vi "PICO-500 Dishwasher 2023.vi"() -> ()   [LabVIEW 2015]
uses:
  <vilib>/userdefined/High Color/IMAQdx.ctl
  <vilib>/express/express signal manip/GetorSetDDTAttributes/Shared VIs/XDimension.ctl
  <vilib>/Utility/file.llb/Write Delimited Spreadsheet (string).vi
  <vilib>/express/express signal manip/GetorSetDDTAttributes/Shared VIs/XDimension Enum to String.vi
  <vilib>/express/express shared/transition.llb/Dynamic To Waveform Array.vi
  <vilib>/express/express signal manip/GetorSetDDTAttributes/Set DDT Attributes/SetT0.vi
  <vilib>/express/express shared/transition.llb/Waveform Array To Dynamic.vi
  <vilib>/express/express signal manip/GetorSetDDTAttributes/Set DDT Attributes/sub Set StartTimeStamp.vi
  <vilib>/FieldPoint/Polymorphic WriteRead.llb/FP WriteRead (Boolean).vi
  <vilib>/measure/mamon.llb/Waveform Peak Detection for 1 Chan.vi
  <vilib>/express/express signal manip/GetorSetDDTAttributes/Set DDT Attributes/Set DDT Properties.xnode
  <vilib>/vision/driver/NI_Vision_Acquisition_Software.lvlib
  <vilib>/express/express signal manip/GetorSetDDTAttributes/Shared VIs/GetSetShared.lvlib
  <vilib>/ptbypt/NI_PtbyPt.lvlib
  <vilib>/Analysis/NI_AALBase.lvlib
  <vilib>/express/express signal manip/GetorSetDDTAttributes/Set DDT Attributes/Set DDT Attributes.lvlib
  <vilib>/measure/NI_MAPro.lvlib
panel:
  out "Current File Path:":path caption="Filename Out"
  in  "Login Tab":enum32{"Login", "Data Aquisition"}(tab)
  in  "Login":bool
  in  "Select Surface":T1(radio)
  in  "Operator Name":string(combo)
  out "Path":path
  out "Live View":bool
  out "System Reset":bool
  in  "DAQ Tab":enum32{"General", "Plots", "Pressure Histogram"}(tab)
  in  "Heat Tape":bool
  in  "PD-25 (Circulation Pump)":bool
  in  "PD-26 (Drain Pump)":bool
  in  "Circulation Mode":bool
  in  "Begin Run":bool
  in  "Return to Login":bool
  out "Surface Selected":string
  in  "Nitrogen Flush Active?":bool
  out "Pressure":dynamicdata(graph)
  out "pH":dynamicdata(graph)
  out "Temperature":dynamicdata(graph)
  out "Heat Tape Circulation Out":dbl
  out "Heat Tape Circulation In":dbl
  out "Pressure Array":dbl[](array[numeric])
  out "Temperature Array":dbl[](array[numeric])
  out "pH Value":dbl
  out "Histogram of Pressure (PT-37)":T2(graph)
  out "Histogram of Pressure (PT-35)":T2(graph)
  out "?":T3(plugin-control)
  in  "Choose camera":T4
  in  "Close Camera":bool
  in  "Shutdown":bool
  out "Program Run-time":string caption="Elapsed Time Text"
  out "Circulation Run-Time":string caption="Elapsed Time Text"
  in  "Emergency Shutdown":bool
  # "PICO-500 Dishwasher DAQ V2.0\nUpdated Jan. 27, 2024"
  # "1. Click the \"Run\" Button - top left white arrow (Rightward facing) \n2. Select or type an operator from the list\n3. Select the Surface that will be cleaned\n4. Click \"Login\""
  # "Adding/Removing Operator:\n\n1. Before selecting \"Run\", right click the \"Operator Name\" string control box and select \"Edit Items\"\n\n2a. To add a new operator, select \"Insert\" and add the operator's name. Select \"ok\" when done.\n\n2b. To remove an operator, select \"Delete\". Select \"ok\" when done.\n\nOperator's name, surface selection, and other operations are recorded in the Activiy_Log.csv file when a new run is initiated."
  # "After Shutdown is complete, Click \"Abort Execution\" (Red Stop Sign Top Left)"
  # "-Nitrogen Flush must be confirmed and latched before \"RUN\" is activated\n-Click \"RUN\" to operate pumps and \"Circulation Mode\"\n-\"RUN\" will also enable live data aquisition and access to the remaining tabs. \"Run\" is active when highlighted green"
  # "Return To the login page. This will reset the current user configurations. \"Run\" must be disabled"
  # "Manual Control (For Adding/Removing cleaing solutions)"
  # "-Heat Tape will automatically turn on after 10 s\n-Heat tape upper limit is set to 200 C\n-Drain pump PD-26 is disabled in this mode\n-PD-25 will automatically run in this mode\n-Lower pressure limit set to 10 psi. When the average pressure reaches this value, the program cycles through the shutdown procedure."
  # "*Heat tape manual control is not recommended. *Heat tape will automatically turn on in circulation mode."
  # "PT-35 [Before Filtration]"
  # "PT-35 (Avg)"
  # "PT-37 [After Filtration]"
  # "PT-37 (Avg)"
  # "Pdiff_35_37 (Avg)"
  # "PT-39 [Pump Inlet]"
  # "PT-39 (Avg)"
  # "TT-38 [Inline Water Temp]"
  # "TT-40 [Ambient Temp]"
  # "TT-41 [Heat Tape Circ. Out]"
  # "TT-42 [Heat Tape Circ. In]"
  # "pH Value"
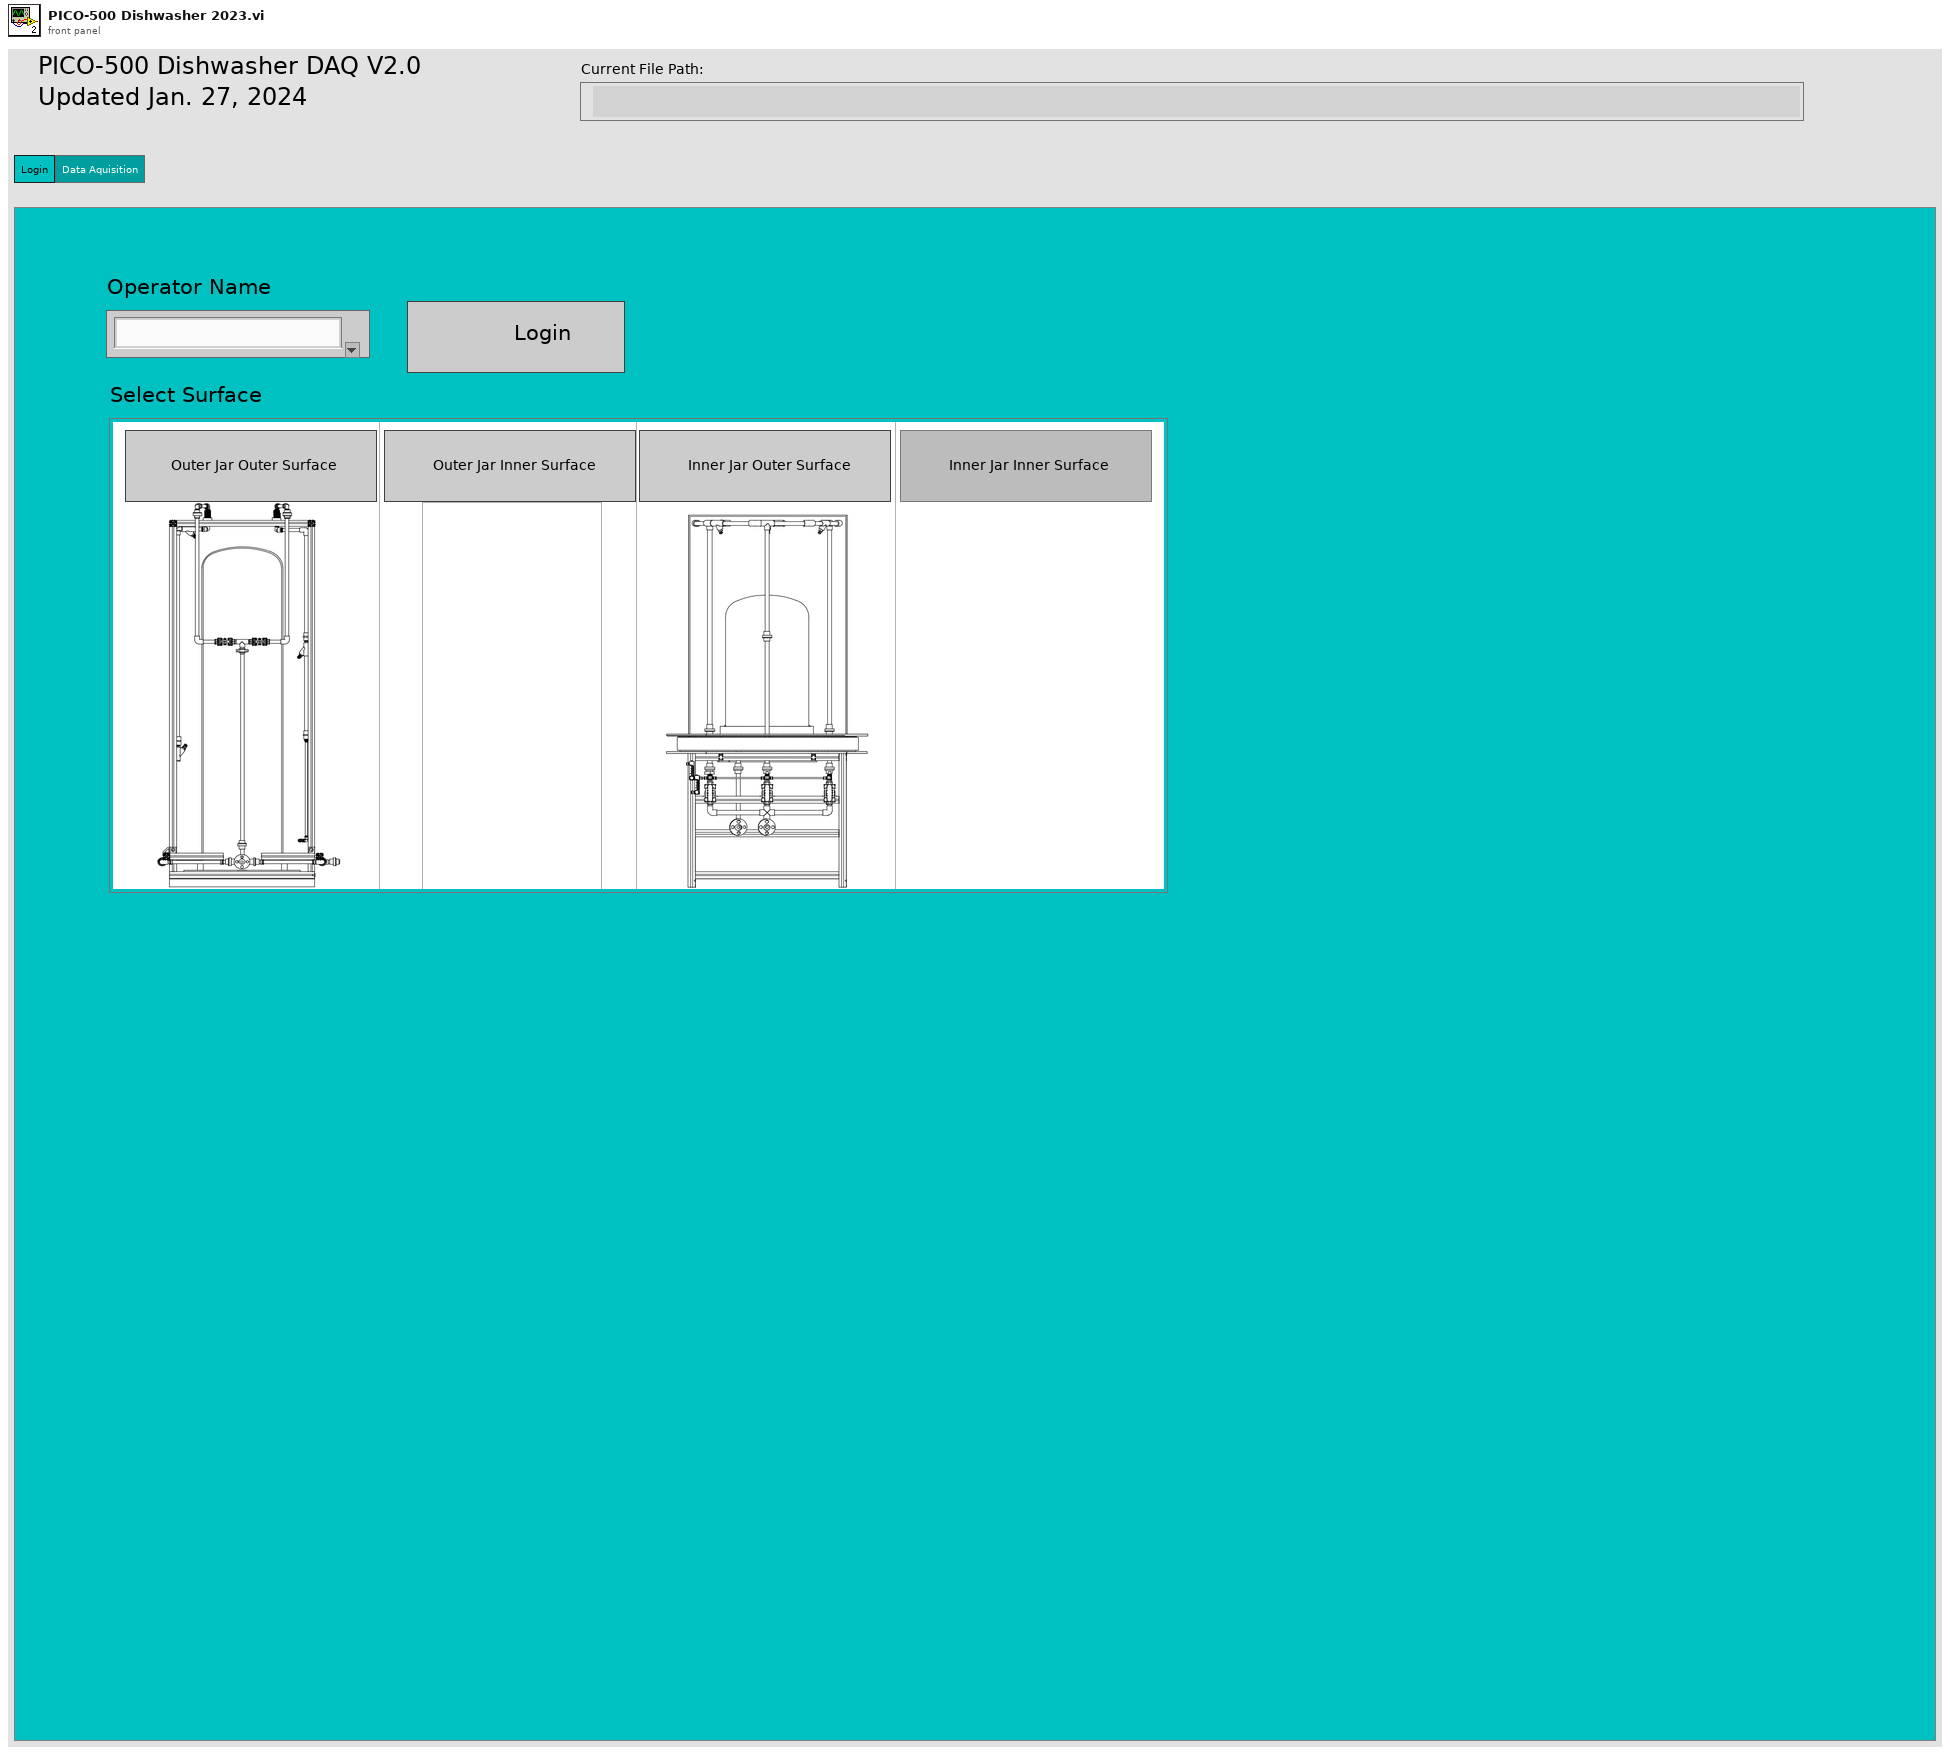
[diagram p1: front panel]
types:
  T1 = enum32{"No Selection", "Inner Jar Inner Surface", "Inner Jar Outer Surface", "Outer Jar Inner Surface", "Outer Jar Outer Surface"}
  T2 = cluster{"X Values":dbl[], "Histogram: h(x)":i32[]}
  T3 = typedef "IMAQ Image.ctl" = refnum<image>
  T4 = typedef "IMAQdx.ctl" = refnum<k21>
  T5 = enum16{"Start", "Login Page", "Go to DAQ", "Run DAQ", "Shutdown Heat Tape", "Shutdown Program", "Stop"}
  T6 = typedef "GetSetShared.lvlib/XDimension.ctl" = enum16{"No Unit [-]", "Time [sec]", "Frequency [Hz]"}
  T7 = cluster{dbl, "mean":dbl, dbl, "mean":dbl, dbl, dbl, "mean":dbl}
  T8 = typedef "Image Type" = u32
  T9 = enum32{"Page Enabled", "Page Disabled", "Page Disabled & Grayed"}
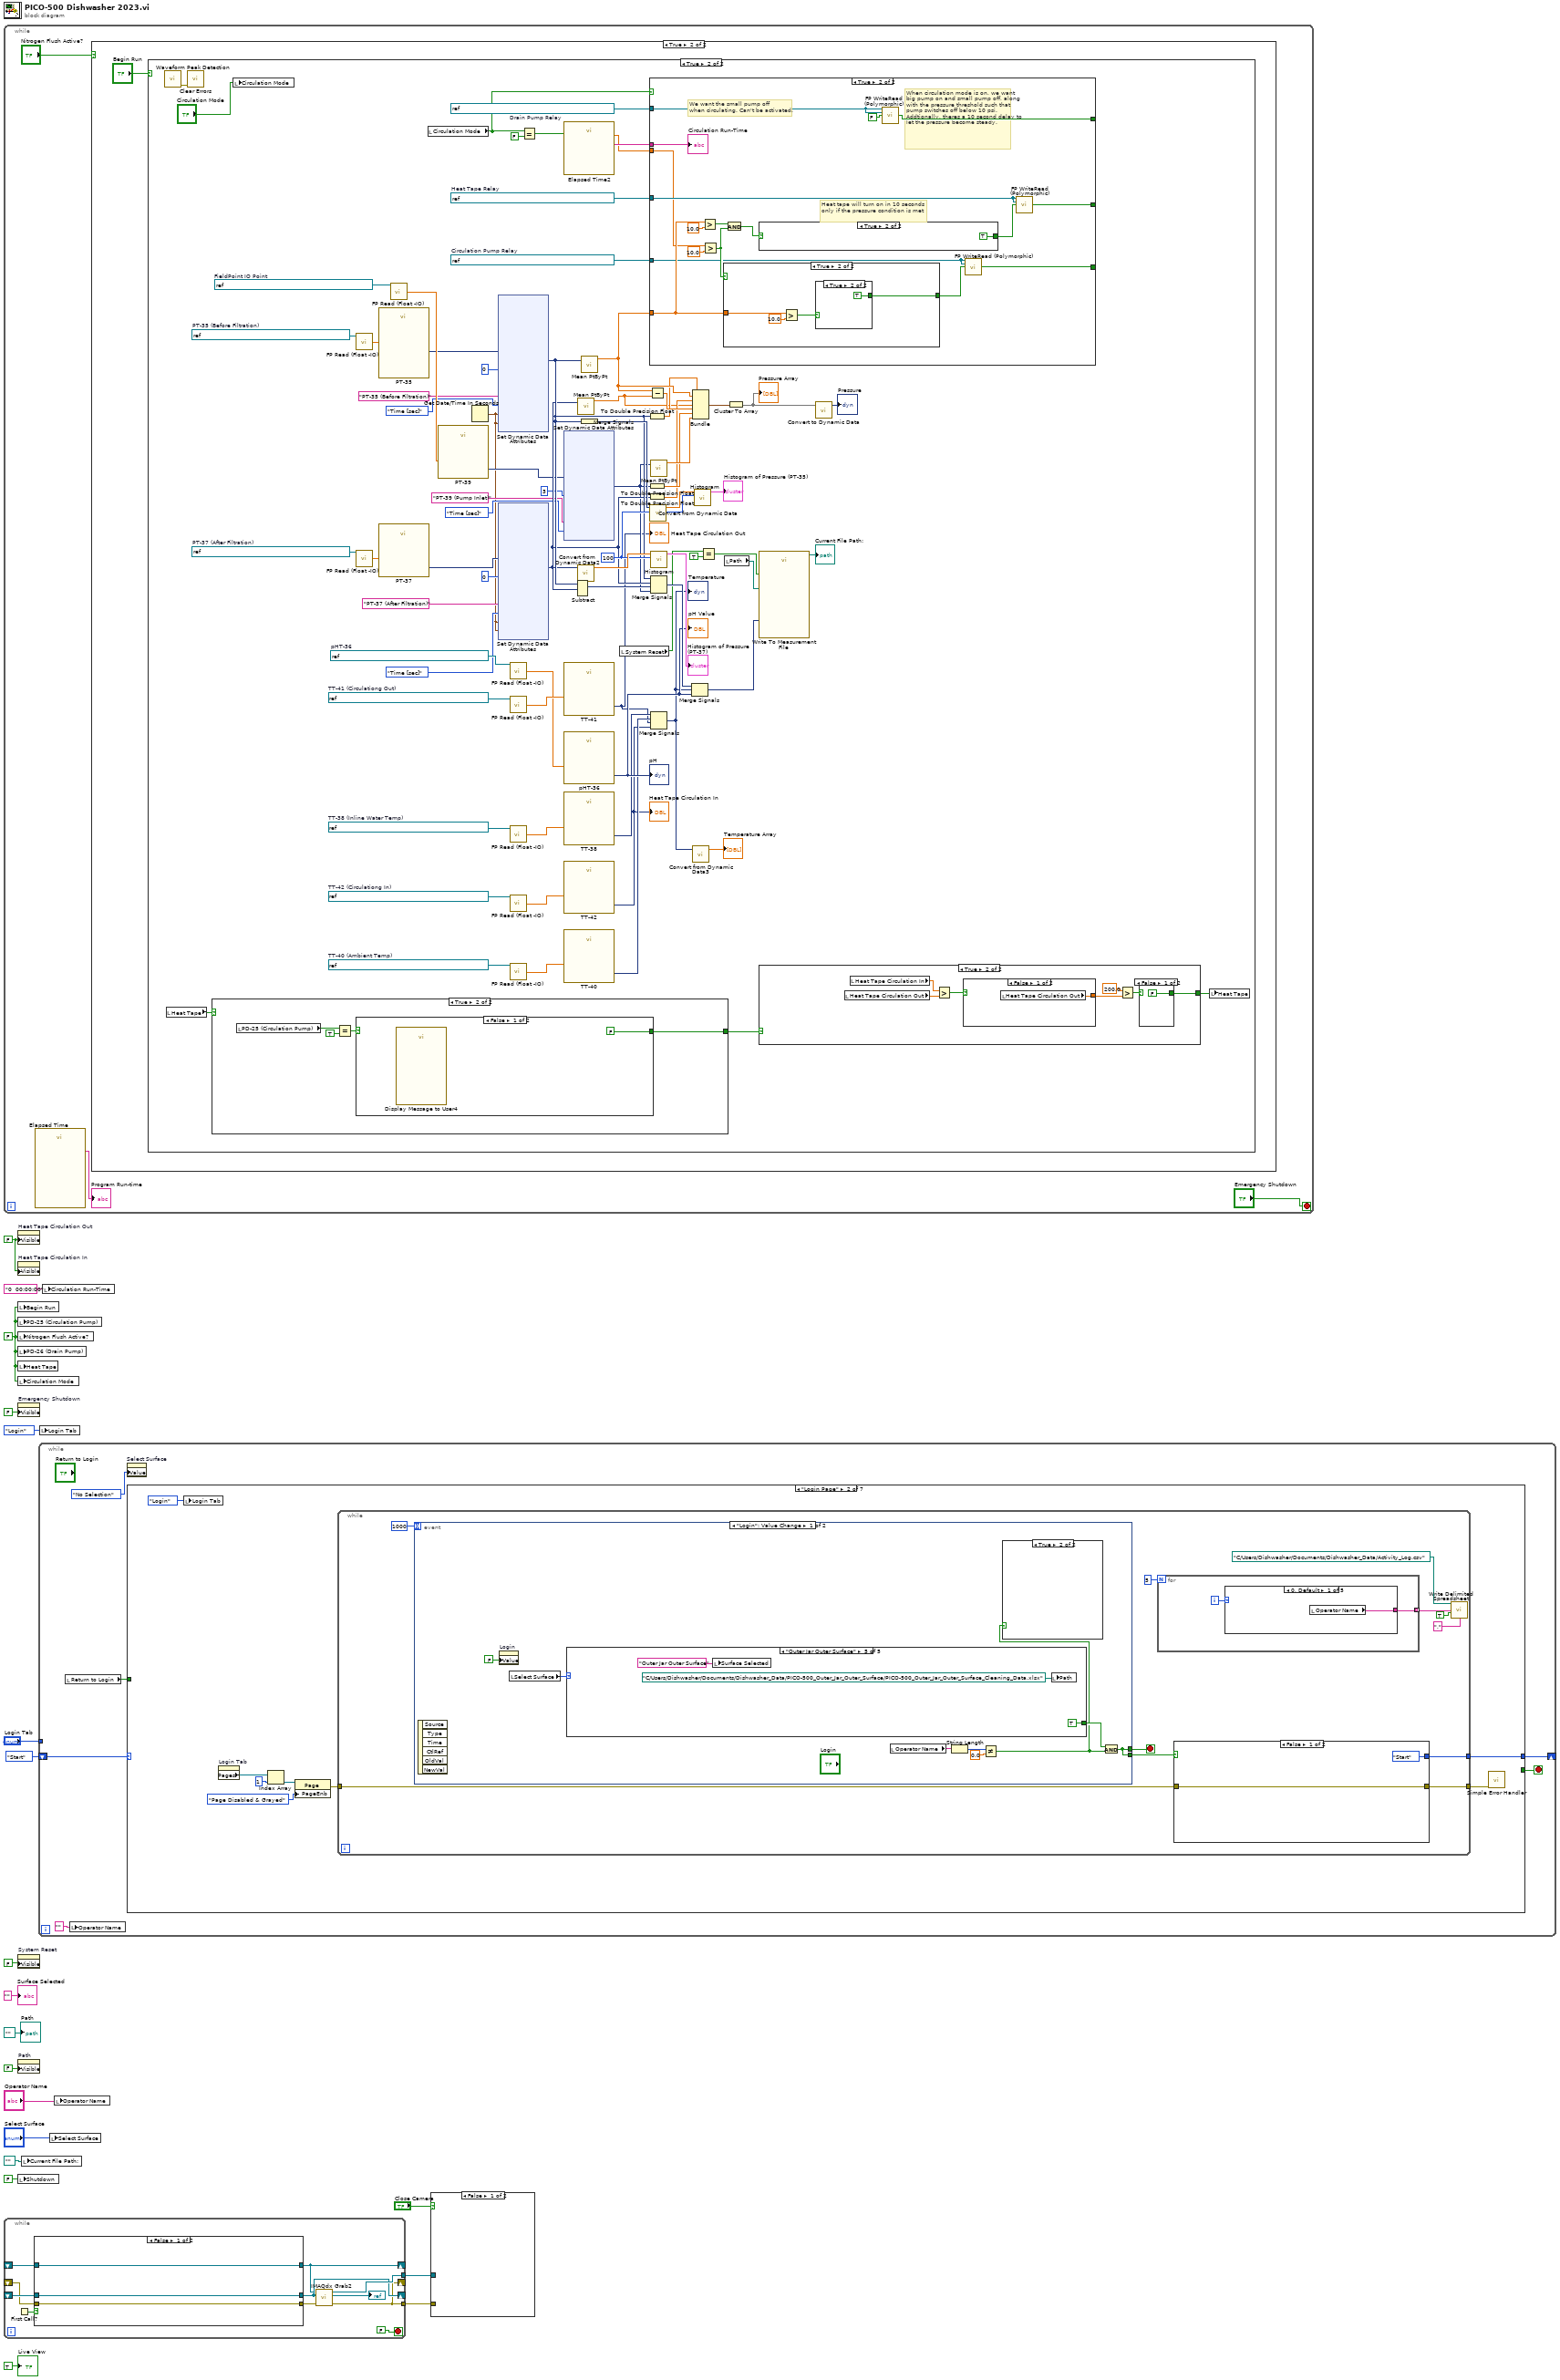
[diagram p0: block diagram]
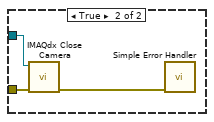
[diagram p2: hidden frame]
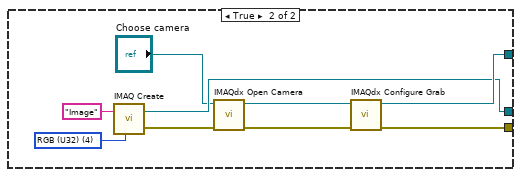
[diagram p3: hidden frame]
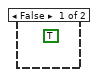
[diagram p5: hidden frame]
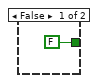
[diagram p6: hidden frame]
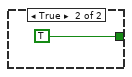
[diagram p7: hidden frame]
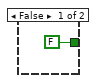
[diagram p8: hidden frame]
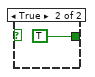
[diagram p9: hidden frame]
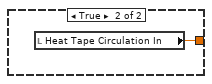
[diagram p10: hidden frame]
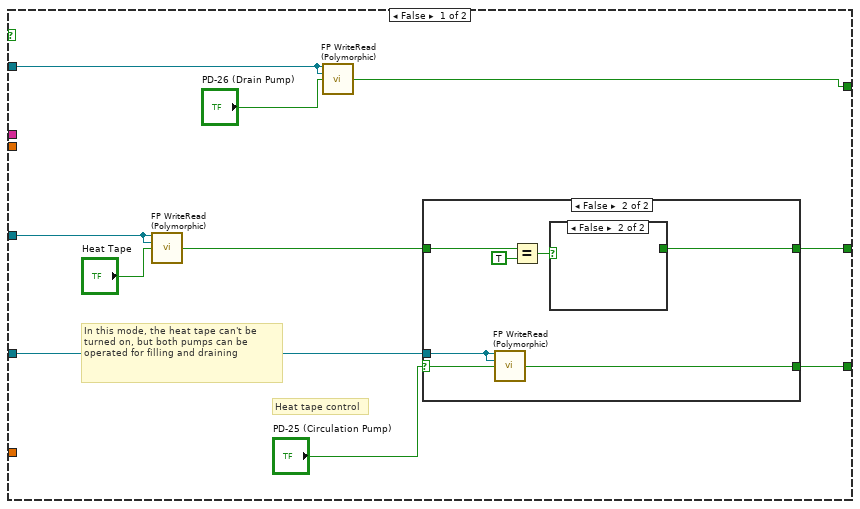
[diagram p11: hidden frame]
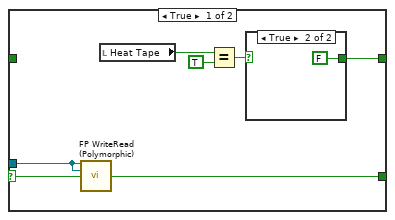
[diagram p12: hidden frame]
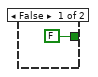
[diagram p13: hidden frame]
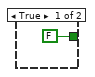
[diagram p14: hidden frame]
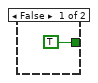
[diagram p15: hidden frame]
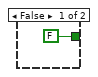
[diagram p16: hidden frame]
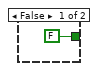
[diagram p17: hidden frame]
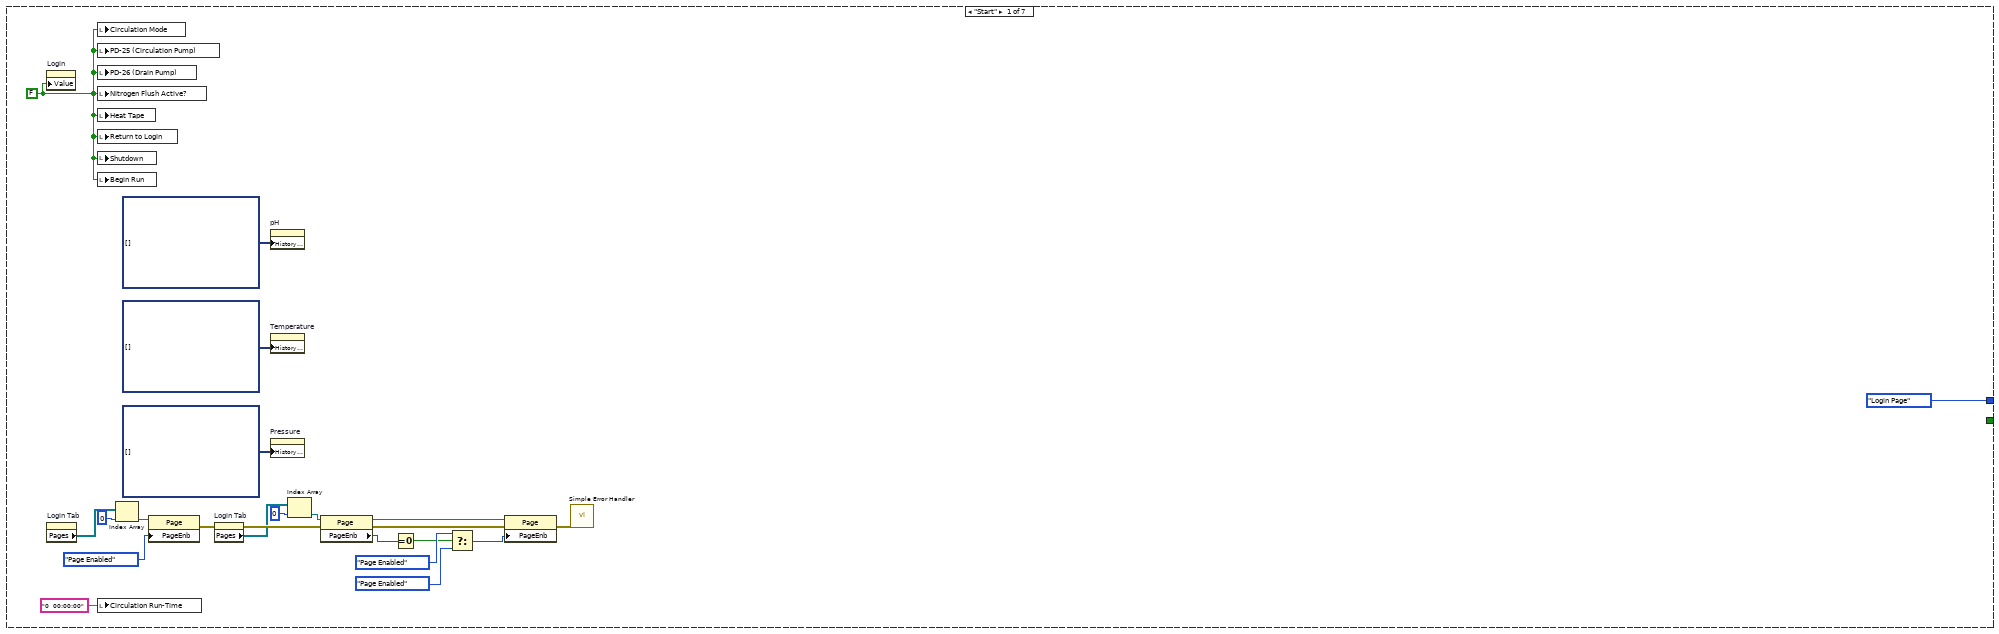
[diagram p18: hidden frame]
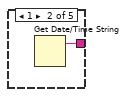
[diagram p19: hidden frame]
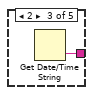
[diagram p20: hidden frame]
diagram:
  w9 = FALSE ("Visible")
  w7 = FALSE
  n1 = while {
    stop <- "Emergency Shutdown" stop-if-true
    n2 = call "Elapsed Time"() -> ("Elapsed Time Text"=→"Program Run-time":string)  [unwired: 12 in, 7 out]
    n3 = case shown="True" "Nitrogen Flush Active?" {
      frame False {
      }
      frame True {
        n4 = case shown="True" "Begin Run" {
          frame False {
            (unwired) TRUE
          }
          frame True {
            w56 = refnum<k21> "FieldPoint\\UofA-CPP-FP\\cFP-RLY-421 @3\\Channel 1"  # Circulation Pump Relay
            w61 = refnum<k21> "FieldPoint\\UofA-CPP-FP\\cFP-RLY-421 @3\\Channel 0"  # Drain Pump Relay
            w54 = refnum<k21> "FieldPoint\\UofA-CPP-FP\\cFP-RLY-421 @3\\Channel 2"  # Heat Tape Relay
            w78 = refnum<k21> "FieldPoint\\UofA-CPP-FP\\cFP-TC-120 @2\\Channel 3"  # TT-41 (Circulationg Out)
            w80 = 100
            w91 = refnum<k21> "FieldPoint\\UofA-CPP-FP\\cFP-TC-120 @2\\Channel 1"  # TT-42 (Circulationg In)
            w92 = refnum<k21> "FieldPoint\\UofA-CPP-FP\\cFP-AI-110 @1\\Channel 2"  # FieldPoint IO Point
            w94 = refnum<k21> "FieldPoint\\UofA-CPP-FP\\cFP-TC-120 @2\\Channel 0"  # TT-40 (Ambient Temp)
            w95 = refnum<k21> "FieldPoint\\UofA-CPP-FP\\cFP-TC-120 @2\\Channel 2"  # TT-38 (Inline Water Temp)
            w96 = refnum<k21> "FieldPoint\\UofA-CPP-FP\\cFP-AI-110 @1\\Channel 3"  # pHT-36
            w97 = refnum<k21> "FieldPoint\\UofA-CPP-FP\\cFP-AI-110 @1\\Channel 1"  # PT-35 (Before Filtration)
            w99 = refnum<k21> "FieldPoint\\UofA-CPP-FP\\cFP-AI-110 @1\\Channel 0"  # PT-37 (After Filtration)
            n5 = call-poly <vilib>:"Waveform Peak Detection.vi"() -> ("error out"=w40:errorcluster)  [unwired: 7 in, 4 out]
            n6 = local read "Heat Tape"() -> (w51:bool)
            n7 = call <vilib>:"Clear Errors.vi"("error in (no error)"=w40) -> ()  [unwired: 5 in, 2 out]
            n8 = case shown="True" w51 {
              tunnel: [FALSE w101] -> w53
              frame False {
              }
              frame True {
                n9 = local read "PD-25 (Circulation Pump)"() -> (w104:bool)
                n10 = Equal?(x=w104, y=TRUE) -> (x = y?=w102:bool)
                n11 = case shown="False" w102 {
                  tunnel: [FALSE TRUE] -> w101
                  frame False {
                    n12 = call "Display Message to User4"() -> ()  [unwired: 10 in, 2 out]
                  }
                  frame True {
                  }
                }
              }
            }
            n13 = local write "Circulation Mode"("Circulation Mode") -> ()
            n14 = call <vilib>:"FP Read (Float -IO).vi"("FieldPoint IO Point In"=w97) -> ("value"=w45:dbl)  [unwired: 11 in, 3 out]
            n15 = call <vilib>:"FP Read (Float -IO).vi"("FieldPoint IO Point In"=w99) -> ("value"=w98:dbl)  [unwired: 11 in, 3 out]
            n16 = call "PT-35"("Signals"=w45) -> ("Scaled Signals"=w43:dynamicdata)  [unwired: 9 in, 1 out]
            n17 = call "PT-37"("Signals"=w98) -> ("Scaled Signals"=w68:dynamicdata)  [unwired: 9 in, 1 out]
            n18 = call <vilib>:"FP Read (Float -IO).vi"("FieldPoint IO Point In"=w92) -> ("value"=w93:dbl)  [unwired: 11 in, 3 out]
            n19 = local read "Circulation Mode"() -> (w58:bool)
            n20 = call "PT-39"("Signals"=w93) -> ("Scaled Signals"=w63:dynamicdata)  [unwired: 9 in, 1 out]
            n21 = Get Date/Time In Seconds() -> (seconds since 1Jan1904=w41:timestamp)
            n22 = xnode "Set Dynamic Data Attributes"("Signals In"=w43, "Signal Index"=0, "Signal Name"="PT-35 (Before Filtration)", "X Dimension"=XDimension."Time [sec]", "Timestamp"=w41, "Start Timestamp"=w41) -> ("Signals Out"=w72:dynamicdata)  [unwired: 1 in, 1 out]
            n23 = xnode "Set Dynamic Data Attributes"("Signals In"=w68, "Signal Index"=0, "Signal Name"="PT-37 (After Filtration)", "X Dimension"=XDimension."Time [sec]", "Timestamp"=w41, "Start Timestamp"=w41) -> ("Signals Out"=w67:dynamicdata)  [unwired: 1 in, 1 out]
            n24 = call <vilib>:"FP Read (Float -IO).vi"("FieldPoint IO Point In"=w96) -> ("value"=w73:dbl)  [unwired: 11 in, 3 out]
            n25 = call <vilib>:"FP Read (Float -IO).vi"("FieldPoint IO Point In"=w78) -> ("value"=w77:dbl)  [unwired: 11 in, 3 out]
            n26 = call <vilib>:"FP Read (Float -IO).vi"("FieldPoint IO Point In"=w95) -> ("value"=w89:dbl)  [unwired: 11 in, 3 out]
            n27 = call <vilib>:"FP Read (Float -IO).vi"("FieldPoint IO Point In"=w91) -> ("value"=w90:dbl)  [unwired: 11 in, 3 out]
            n28 = call <vilib>:"FP Read (Float -IO).vi"("FieldPoint IO Point In"=w94) -> ("value"=w88:dbl)  [unwired: 11 in, 3 out]
            n29 = Equal?(x=w58, y=FALSE) -> (x = y?=w59:bool)
            n30 = call "Elapsed Time2"("Reset"=w59) -> ("Elapsed Time (s)"=w50:dbl, "Elapsed Time Text"=w55:string)  [unwired: 11 in, 6 out]
            n31 = xnode "Set Dynamic Data Attributes"("Signals In"=w63, "Signal Index"=3, "Signal Name"="PT-39 (Pump Inlet)", "X Dimension"=XDimension."Time [sec]") -> ("Signals Out"=w62:dynamicdata)  [unwired: 1 in, 1 out]
            n32 = call "TT-41"("Signals"=w77) -> ("Scaled Signals"=w32:dynamicdata)  [unwired: 9 in, 1 out]
            "Heat Tape Circulation Out" <- w32
            n33 = call "pHT-36"("Signals"=w73) -> ("Scaled Signals"=w81:dynamicdata)  [unwired: 9 in, 1 out]
            "pH" <- w81
            "pH Value" <- w81
            n34 = call "TT-38"("Signals"=w89) -> ("Scaled Signals"=w34:dynamicdata)  [unwired: 9 in, 1 out]
            n35 = call "TT-42"("Signals"=w90) -> ("Scaled Signals"=w31:dynamicdata)  [unwired: 9 in, 1 out]
            "Heat Tape Circulation In" <- w31
            n36 = call "TT-40"("Signals"=w88) -> ("Scaled Signals"=w33:dynamicdata)  [unwired: 9 in, 1 out]
            n37 = Subtract(1:w67, 2:w72) -> (0:w79:dynamicdata)  [unwired: 1 in, 1 out]
            n38 = call "Convert from Dynamic Data2"("Dynamic Data Type"=w67) -> ("Array"=w84:dbl[])  [unwired: 3 in]
            n39 = call <vilib>:"Mean PtByPt.vi"("x"=w67) -> ("mean"=w24:dbl)  [unwired: 3 in, 1 out]
            n40 = call <vilib>:"Mean PtByPt.vi"("x"=w72) -> ("mean"=w29:dbl)  [unwired: 3 in, 1 out]
            n41 = Merge Signals(w72) -> (w85:dynamicdata)
            n42 = local read "System Reset"() -> (w48:bool)
            n43 = case shown="True" w58 {
              tunnel: w29 -> [_ w154]
              tunnel: [w127 w161] -> _
              tunnel: [w124 w148] -> _
              tunnel: w61 -> [w125 w159]
              tunnel: w56 -> [w123 w152]
              tunnel: w54 -> [w120 w153]
              tunnel: [w122 w147] -> _
              tunnel: w50 -> [_ w149]
              tunnel: w55 -> [_ w146]
              frame False {
                # "Heat tape control"
                # "In this mode, the heat tape can't be turned on, but both pumps can be operated for filling and draining"
                n44 = call-poly <vilib>:"FP WriteRead (Polymorphic).vi"("FieldPoint Write Point"=w120, "FieldPoint Read Point"=w120, "value in"="Heat Tape") -> ("value out"=w119:bool)  [unwired: 10 in, 2 out]
                n45 = call-poly <vilib>:"FP WriteRead (Polymorphic).vi"("FieldPoint Write Point"=w125, "FieldPoint Read Point"=w125, "value in"="PD-26 (Drain Pump)") -> ("value out"=w127:bool)  [unwired: 10 in, 2 out]
                n46 = case shown="False" "PD-25 (Circulation Pump)" {
                  selector: "PD-25 (Circulation Pump)" -> [w134 w141]
                  tunnel: [w129 w142] -> w124
                  tunnel: w123 -> [w135 w139]
                  tunnel: [w133 w140] -> w122
                  tunnel: w119 -> [_ w138]
                  frame True {
                    n47 = call-poly <vilib>:"FP WriteRead (Polymorphic).vi"("FieldPoint Write Point"=w135, "FieldPoint Read Point"=w135, "value in"=w134) -> ("value out"=w133:bool)  [unwired: 10 in, 2 out]
                    n48 = local read "Heat Tape"() -> (w132:bool)
                    n49 = Equal?(x=w132, y=TRUE) -> (x = y?=w130:bool)
                    n50 = case shown="True" w130 {
                      tunnel: [FALSE FALSE] -> w129
                      frame False {
                      }
                      frame True {
                      }
                    }
                  }
                  frame False {
                    n51 = call-poly <vilib>:"FP WriteRead (Polymorphic).vi"("FieldPoint Write Point"=w139, "FieldPoint Read Point"=w139, "value in"=w141) -> ("value out"=w140:bool)  [unwired: 10 in, 2 out]
                    n52 = Equal?(x=w138, y=TRUE) -> (x = y?=w143:bool)
                    n53 = case shown="False" w143 {
                      tunnel: [FALSE _] -> w142
                      frame True {
                      }
                      frame False {
                      }
                    }
                  }
                }
              }
              frame True {
                # "Heat tape will turn on in 10 seconds only if the pressure condition is met"
                # "We want the small pump off\nwhen circulating. Can't be activated."
                # "When circulation mode is on, we want big pump on and small pump off, along with the pressure threshold such that pump switches off below 10 psi. Addtionally, theres a 10 second delay to let the pressure become steady."
                n54 = Greater?(x=w154, y=10.0 ("Pressure threshold ijo")) -> (0:w157:bool)
                n55 = Greater?(x=w149, y=10.0 ("Pressure threshold ijo")) -> (0:w155:bool)
                n56 = case shown="True" w155 {
                  tunnel: w154 -> [_ w166]
                  tunnel: [TRUE w164] -> w150
                  frame False {
                  }
                  frame True {
                    n57 = Greater?(x=w166, y=10.0 ("Pressure threshold ijo")) -> (0:w165:bool)
                    n58 = case shown="True" w165 {
                      tunnel: [FALSE TRUE] -> w164
                      frame False {
                      }
                      frame True {
                      }
                    }
                  }
                }
                n59 = And(x=w157, y=w155) -> (x .and. y?=w156:bool)
                n60 = case shown="True" w156 {
                  tunnel: [FALSE TRUE] -> w151
                  frame False {
                  }
                  frame True {
                  }
                }
                n61 = call-poly <vilib>:"FP WriteRead (Polymorphic).vi"("FieldPoint Write Point"=w159, "FieldPoint Read Point"=w159, "value in"=FALSE) -> ("value out"=w161:bool)  [unwired: 10 in, 2 out]
                n62 = call-poly <vilib>:"FP WriteRead (Polymorphic).vi"("FieldPoint Write Point"=w152, "FieldPoint Read Point"=w152, "value in"=w150) -> ("value out"=w147:bool)  [unwired: 10 in, 2 out]
                n63 = call-poly <vilib>:"FP WriteRead (Polymorphic).vi"("FieldPoint Write Point"=w153, "FieldPoint Read Point"=w153, "value in"=w151) -> ("value out"=w148:bool)  [unwired: 10 in, 2 out]
                "Circulation Run-Time" <- w146
              }
            }
            n64 = Subtract(x=w29, y=w24) -> (x-y=w30:dbl)
            n65 = To Double Precision Float(number=w72) -> (double precision float=w28:dbl)
            n66 = To Double Precision Float(number=w62) -> (double precision float=w26:dbl)
            n67 = To Double Precision Float(number=w67) -> (double precision float=w25:dbl)
            n68 = call "Convert from Dynamic Data"("Dynamic Data Type"=w85) -> ("Array"=w86:dbl[])  [unwired: 3 in]
            n69 = call <vilib>:"Mean PtByPt.vi"("x"=w62) -> ("mean"=w27:dbl)  [unwired: 3 in, 1 out]
            n70 = Merge Signals(w72, w67, w79, w62) -> (w82:dynamicdata)
            n71 = call <vilib>:"Histogram.vi"("intervals"=w80, "X"=w84) -> ("Histogram Graph"=→"Histogram of Pressure (PT-37)":T2)  [unwired: 6 in, 3 out]
            n72 = Merge Signals(w34, w33, w32, w31) -> (w35:dynamicdata)
            "Temperature" <- w35
            n73 = Merge Signals(w82, w35, w81) -> (w44:dynamicdata)
            n74 = Bundle(w28, "mean"=w29, w25, "mean"=w24, w30, w26, "mean"=w27) -> (w39:T7)  [unwired: 1 in]
            n75 = call "Convert from Dynamic Data3"("Dynamic Data Type"=w35) -> ("Array"=→"Temperature Array":dbl[])  [unwired: 3 in]
            n76 = call <vilib>:"Histogram.vi"("intervals"=w80, "X"=w86) -> ("Histogram Graph"=→"Histogram of Pressure (PT-35)":T2)  [unwired: 6 in, 3 out]
            n77 = Equal?(x=w48, y=TRUE) -> (x = y?=w46:bool)
            n78 = local read "Path"() -> (w42:path)
            n79 = Cluster To Array(cluster=w39) -> (array=w38:dbl[])
            "Pressure Array" <- w38
            n80 = call "Write To Measurement File"("Signals"=w44, "new_file"=w46, "Filename"=w42) -> ("Filename Out"=→"Current File Path:":path)  [unwired: 14 in, 2 out]
            n81 = case shown="True" w53 {
              tunnel: [FALSE w114] -> w52
              frame False {
              }
              frame True {
                n82 = local read "Heat Tape Circulation Out"() -> (w109:dbl)
                n83 = local read "Heat Tape Circulation In"() -> (w110:dbl)
                n84 = Greater?(x=w110, y=w109) -> (0:w113:bool)
                n85 = case shown="False" w113 {
                  tunnel: [w117 w118] -> w108
                  frame False {
                    n86 = local read "Heat Tape Circulation Out"() -> (w117:dbl)
                  }
                  frame True {
                    n87 = local read "Heat Tape Circulation In"() -> (w118:dbl)
                  }
                }
                n88 = Greater?(x=200.0, y=w108) -> (0:w112:bool)
                n89 = case shown="False" w112 {
                  tunnel: [FALSE TRUE] -> w114
                  frame False {
                  }
                  frame True {
                  }
                }
              }
            }
            n90 = call "Convert to Dynamic Data"("Array"=w38) -> ("Dynamic Data Type"=→"Pressure":dynamicdata)  [unwired: 3 in]
            n91 = local write "Heat Tape"(w52) -> ()
          }
        }
      }
    }
  }
  n92 = while {
    tunnel: [w250] -> w4
    tunnel: [w243] -> w3
    shift-right: [w247] -> _
    shift-left: _ -> [w246]
    shift-right: [w245] -> _
    shift-left: _ -> [w244]
    shift-right: [w243] -> _
    shift-left: _ -> [w242]
    stop <- FALSE stop-if-true
    n93 = First Call?() -> (First Call?: T/F=w248:bool)
    n94 = case shown="False" w248 {
      tunnel: [w252 w261] -> w245
      tunnel: [w251 w259] -> w249
      tunnel: [w253 w256] -> w247
      tunnel: w246 -> [w253 _]
      tunnel: w244 -> [w252 _]
      tunnel: w242 -> [w251 _]
      frame False {
      }
      frame True {
        w257 = T8 4 items=["Grayscale (U8)", "Grayscale (I16)", "Grayscale (SGL)", "Complex (CSG)", "RGB (U32)", "HSL (U32)", "RGB (U64)", "Grayscale (U16)"] ("Image Type")
        n95 = call "IMAQ Create"("Image Name"="Image", "Image Type"=w257) -> ("New Image"=w256:T3, "error out"=w255:errorcluster)  [unwired: 3 in]
        n96 = call <vilib>:"IMAQdx Open Camera.vi"("error in"=w255, "Session In"="Choose camera") -> ("error out"=w260:errorcluster, "Session Out"=w262:T4)  [unwired: 8 in]
        n97 = call <vilib>:"IMAQdx Configure Grab.vi"("error in"=w260, "Session In"=w262) -> ("error out"=w259:errorcluster, "Session Out"=w261:T4)  [unwired: 8 in]
      }
    }
    n98 = call <vilib>:"IMAQdx Grab2.vi"("error in"=w249, "Image In"=w247, "Session In"=w245) -> ("error out"=w243:errorcluster, "Image Out"=→"?":T3, "Session Out"=w250:T4)  [unwired: 5 in, 1 out]
  }
  n99 = property on="Heat Tape Circulation Out" class="DigNum (strict)"("Visible"=w9) -> ()  [unwired: 2 in, 2 out]
  n100 = property on="Heat Tape Circulation In" class="DigNum (strict)"("Visible"=w9) -> ()  [unwired: 2 in, 2 out]
  n101 = local write "Begin Run"(w7) -> ()
  n102 = local write "PD-25 (Circulation Pump)"(w7) -> ()
  n103 = local write "Nitrogen Flush Active?"(w7) -> ()
  n104 = local write "PD-26 (Drain Pump)"(w7) -> ()
  n105 = local write "Heat Tape"(w7) -> ()
  n106 = local write "Circulation Mode"(w7) -> ()
  n107 = property on="Emergency Shutdown" class="Bool (strict)"("Visible"=FALSE) -> ()  [unwired: 2 in, 2 out]
  n108 = property on="System Reset" class="Bool (strict)"("Visible"=FALSE) -> ()  [unwired: 2 in, 2 out]
  n109 = property on="Path" class="Path"("Visible"=FALSE) -> ()  [unwired: 2 in, 2 out]
  n110 = local write "Shutdown"(FALSE) -> ()
  n111 = local write "Current File Path:"(path "" ("Current File Path:")) -> ()
  n112 = while {
    shift-right: [w267] -> _
    shift-left: T5."Start" -> [w268]
    tunnel: "Login Tab" -> [_]
    stop <- w266 stop-if-true
    n113 = local read "Return to Login"() -> (w263:bool)
    n114 = local write "Operator Name"("") -> ()
    n115 = property on="Select Surface" class="RadioBtnsControl (strict)"("Value"=T1."No Selection" ("Select Surface")) -> ()  [unwired: 2 in, 2 out]
    n116 = case shown="\"Login Page\"" w268 {
      tunnel: [T5."Login Page" w293 T5."Run DAQ" w388 T5."Shutdown Program" w411 T5."Stop"] -> w267
      tunnel: [_ _ _ _ _ _ TRUE] -> w266
      tunnel: w263 -> [_ _ _ w387 _ _ _]
      frame "Start" {
        w271 = FALSE ("Begin Run")
        n117 = property on="Login" class="Bool (strict)"("Value"=w271) -> ()  [unwired: 2 in, 2 out]
        n118 = property on="Login Tab" class="TabCtl (strict)"() -> ("Pages"=w288:refnum<vi>[])  [unwired: 2 in, 2 out]
        n119 = local write "Circulation Mode"(w271) -> ()
        n120 = local write "PD-25 (Circulation Pump)"(w271) -> ()
        n121 = local write "PD-26 (Drain Pump)"(w271) -> ()
        n122 = local write "Nitrogen Flush Active?"(w271) -> ()
        n123 = local write "Heat Tape"(w271) -> ()
        n124 = local write "Return to Login"(w271) -> ()
        n125 = local write "Shutdown"(w271) -> ()
        n126 = local write "Begin Run"(w271) -> ()
        n127 = local write "Circulation Run-Time"("0  00:00:00" ("Circulation Run-Time")) -> ()
        n128 = Index Array(array=w288, index=0) -> (element=w290:refnum<vi>)
        n129 = property class="Page"(reference=w290, "PageEnb"=T9."Page Enabled" ("Page Enabled State")) -> (error out=w276:errorcluster)  [unwired: 1 in, 1 out]
        n130 = property on="Login Tab" class="TabCtl (strict)"(error in=w276) -> (error out=w286:errorcluster, "Pages"=w277:refnum<vi>[])  [unwired: 1 in, 1 out]
        n131 = property on="pH" class="WFChart (strict)"("History Data"=dynamicdata[] []) -> ()  [unwired: 2 in, 2 out]
        n132 = property on="Temperature" class="WFChart (strict)"("History Data"=dynamicdata[] []) -> ()  [unwired: 2 in, 2 out]
        n133 = property on="Pressure" class="WFChart (strict)"("History Data"=dynamicdata[] []) -> ()  [unwired: 2 in, 2 out]
        n134 = Index Array(array=w277, index=0) -> (element=w279:refnum<vi>)
        n135 = property class="Page"(reference=w279, error in=w286) -> (reference out=w280:refnum<vi>, error out=w287:errorcluster, "PageEnb"=w281:T9)
        n136 = Equal To 0?(x=w281) -> (x = 0?=w282:bool)
        n137 = Select(t=T9."Page Enabled" ("Page Enabled State"), s=w282, f=T9."Page Enabled" ("Page Enabled State")) -> (s? t:f=w285:T9)
        n138 = property class="Page"(reference=w280, error in=w287, "PageEnb"=w285) -> (error out=w275:errorcluster)  [unwired: 1 out]
        n139 = call <vilib>:"Simple Error Handler.vi"("error in (no error)"=w275) -> ()  [unwired: 4 in, 5 out]
      }
      frame "Login Page" {
        n140 = local write "Login Tab"(enum32{"Login", "Data Aquisition"}."Login" ("Tab Control 3")) -> ()
        n141 = property on="Login Tab" class="TabCtl (strict)"() -> ("Pages"=w294:refnum<vi>[])  [unwired: 2 in, 2 out]
        n142 = Index Array(array=w294, index=1) -> (element=w296:refnum<vi>)
        n143 = property class="Page"(reference=w296, "PageEnb"=T9."Page Disabled & Grayed" ("Page Enabled State")) -> (error out=w298:errorcluster)  [unwired: 1 in, 1 out]
        n144 = while {
          tunnel: w298 -> [w309]
          tunnel: [w308] -> w299
          tunnel: [w306] -> w293
          stop <- w310 stop-if-true
          n145 = event shown="[0] \"Login\": Value Change" {
            selector: _ -> [_ _]
            dyn-events: _ -> [_ _]
            timeout: 1000 -> [_ _]
            tunnel: [w339 _] -> w310
            tunnel: [w339 _] -> w307
            event "Login": Value Change {
              n146 = event-data() -> ()  [unwired: 1 in, 6 out]
              n147 = property on="Login" class="Bool (strict)"("Value"=FALSE ("Login")) -> ()  [unwired: 2 in, 2 out]
              n148 = local read "Select Surface"() -> (w341:T1)
              n149 = case shown="\"Outer Jar Outer Surface\"" w341 {
                tunnel: [FALSE TRUE TRUE TRUE TRUE] -> w340
                frame "No Selection", Default {
                  n150 = call "Display Message to User3"() -> ()  [unwired: 10 in, 2 out]
                }
                frame "Inner Jar Inner Surface" {
                  n151 = local write "Surface Selected"("Inner Jar Inner Surface") -> ()
                  n152 = local write "Path"(path "C:/Users/Dishwasher/Documents/Dishwasher_Data/PICO-500_Inner_Jar_Inner_Surface/PICO-500_Inner_Jar_Inner_Surface_Cleaning_Data.xlsx" ("Path")) -> ()
                }
                frame "Inner Jar Outer Surface" {
                  n153 = local write "Surface Selected"("Inner Jar Outer Surface") -> ()
                  n154 = local write "Path"(path "C:/Users/Dishwasher/Documents/Dishwasher_Data/PICO-500_Inner_Jar_Outer_Surface/PICO-500_Inner_Jar_Outer_Surface_Cleaning_Data.xlsx" ("Path")) -> ()
                }
                frame "Outer Jar Inner Surface" {
                  n155 = local write "Surface Selected"("Outer Jar Inner Surface") -> ()
                  n156 = local write "Path"(path "C:/Users/Dishwasher/Documents/Dishwasher_Data/PICO-500_Outer_Jar_Inner_Surface/PICO-500_Outer_Jar_Inner_Surface_Cleaning_Data.xlsx" ("Path")) -> ()
                }
                frame "Outer Jar Outer Surface" {
                  n157 = local write "Surface Selected"("Outer Jar Outer Surface") -> ()
                  n158 = local write "Path"(path "C:/Users/Dishwasher/Documents/Dishwasher_Data/PICO-500_Outer_Jar_Outer_Surface/PICO-500_Outer_Jar_Outer_Surface_Cleaning_Data.xlsx" ("Path")) -> ()
                }
              }
              n159 = local read "Operator Name"() -> (w335:string)
              n160 = String Length(string=w335) -> (length=w337:i32)
              n161 = Not Equal?(x=w337, y=0.0) -> (x != y?=w336:bool)
              n162 = case shown="True" w336 {
                frame False {
                  n163 = call "Display Message to User2"() -> ()  [unwired: 10 in, 2 out]
                }
                frame True {
                }
              }
              n164 = And(x=w340, y=w336) -> (x .and. y?=w339:bool)
            }
            event Timeout {
              n165 = event-data() -> ()  [unwired: 1 in, 3 out]
            }
          }
          n166 = for {
            N: 5 -> [_]
            tunnel: [w311] -> w302 mode=indexing
            i -> [w312]
            n167 = case shown="0, Default" w312 {
              tunnel: [w313 w314 w315 w316 "Starting the LabVIEW program"] -> w311
              frame 0, Default {
                n168 = local read "Operator Name"() -> (w313:string)
              }
              frame 1 {
                n169 = Get Date/Time String() -> (date string=w314:string)  [unwired: 3 in, 1 out]
              }
              frame 2 {
                n170 = Get Date/Time String() -> (time string=w315:string)  [unwired: 3 in, 1 out]
              }
              frame 4 {
                n171 = local read "Surface Selected"() -> (w316:string)
              }
              frame 3 {
              }
            }
          }
          n172 = case shown="False" w307 {
            tunnel: w309 -> [w319 w331]
            tunnel: [w319 w323] -> w308
            tunnel: [T5."Start" T5."Go to DAQ"] -> w306
            frame False {
            }
            frame True {
              n173 = property on="Login Tab" class="TabCtl (strict)"(error in=w331) -> (error out=w322:errorcluster, "Pages"=w333:refnum<vi>[])  [unwired: 1 in, 1 out]
              n174 = Index Array(array=w333, index=1) -> (element=w330:refnum<vi>)
              n175 = property class="Page"(reference=w330, error in=w322) -> (reference out=w329:refnum<vi>, error out=w321:errorcluster, "PageEnb"=w328:T9)
              n176 = Equal To 0?(x=w328) -> (x = 0?=w327:bool)
              n177 = Select(t=T9."Page Disabled & Grayed" ("Page Enabled State"), s=w327, f=T9."Page Enabled" ("Page Enabled State")) -> (s? t:f=w324:T9)
              n178 = property class="Page"(reference=w329, error in=w321, "PageEnb"=w324) -> (error out=w323:errorcluster)  [unwired: 1 out]
            }
          }
          n179 = call-poly <vilib>:"Write Delimited Spreadsheet.vi"("file path (dialog if empty)"=path "C:/Users/Dishwasher/Documents/Dishwasher_Data/Activity_Log.csv", "1D data"=w302, "append to file? (F)"=TRUE, "delimiter (\\t)"="," ("delimiter (\\t)")) -> ()  [unwired: 10 in, 2 out]
        }
        n180 = call <vilib>:"Simple Error Handler.vi"("error in (no error)"=w299) -> ()  [unwired: 4 in, 5 out]
      }
      frame "Go to DAQ" {
        n181 = Wait (ms)(milliseconds to wait=u32 50) -> ()  [unwired: 1 out]
        n182 = local write "DAQ Tab"(enum32{"General", "Plots", "Pressure Histogram"}."General" ("DAQ Tab")) -> ()
        n183 = property on="Login Tab" class="TabCtl (strict)"() -> ("Pages"=w362:refnum<vi>[])  [unwired: 2 in, 2 out]
        n184 = local write "Login Tab"(enum32{"Login", "Data Aquisition"}."Data Aquisition" ("Tab Control 3")) -> ()
        n185 = Index Array(array=w362, index=0) -> (element=w364:refnum<vi>)
        n186 = local read "Shutdown"() -> (w359:bool)
        n187 = property class="Page"(reference=w364, "PageEnb"=T9."Page Disabled & Grayed" ("Page Enabled State")) -> (error out=w360:errorcluster)  [unwired: 1 in, 1 out]
        n188 = case shown="False" w359 {
          tunnel: [w366 w368] -> w361
          tunnel: w360 -> [w366 w367]
          frame False {
          }
          frame True {
            n189 = property on="Login Tab" class="TabCtl (strict)"(error in=w367) -> (error out=w378:errorcluster, "Pages"=w369:refnum<vi>[])  [unwired: 1 in, 1 out]
            n190 = Index Array(array=w369, index=0) -> (element=w371:refnum<vi>)
            n191 = property class="Page"(reference=w371, error in=w378) -> (reference out=w372:refnum<vi>, error out=w379:errorcluster, "PageEnb"=w373:T9)
            n192 = Equal To 0?(x=w373) -> (x = 0?=w374:bool)
            n193 = Select(t=T9."Page Disabled & Grayed" ("Page Enabled State"), s=w374, f=T9."Page Enabled" ("Page Enabled State")) -> (s? t:f=w377:T9)
            n194 = property class="Page"(reference=w372, error in=w379, "PageEnb"=w377) -> (error out=w368:errorcluster)  [unwired: 1 out]
          }
        }
        n195 = call <vilib>:"Simple Error Handler.vi"("error in (no error)"=w361) -> ()  [unwired: 4 in, 5 out]
      }
      frame "Run DAQ" {
        n196 = case shown="False" w387 {
          tunnel: [w392 w400] -> w388
          frame False {
            n197 = local read "Begin Run"() -> (w391:bool)
            n198 = case shown="True" w391 {
              tunnel: [T5."Go to DAQ" T5."Run DAQ"] -> w394
              frame False {
                n199 = local write "System Reset"(TRUE) -> ()
              }
              frame True {
                n200 = local write "System Reset"(FALSE) -> ()
              }
            }
            n201 = Select(t=T5."Shutdown Heat Tape", s="Shutdown", f=w394) -> (s? t:f=w392:T5)
          }
          frame True {
            n202 = local read "Begin Run"() -> (w399:bool)
            n203 = case shown="False" w399 {
              tunnel: [T5."Start" T5."Run DAQ"] -> w400
              frame False {
                n204 = local write "Heat Tape"(FALSE) -> ()
                n205 = local write "Circulation Mode"(FALSE) -> ()
                n206 = local write "PD-25 (Circulation Pump)"(FALSE) -> ()
                n207 = local write "PD-26 (Drain Pump)"(FALSE) -> ()
                "System Reset" <- FALSE
              }
              frame True {
                n208 = call "Display Message to User"() -> ()  [unwired: 10 in, 2 out]
              }
            }
          }
        }
        n209 = local read "Nitrogen Flush Active?"() -> (w386:bool)
        n210 = local read "Begin Run"() -> (w384:bool)
        n211 = Equal?(x=w386, y=FALSE) -> (x = y?=w382:bool)
        n212 = Equal?(x=w384, y=TRUE) -> (x = y?=w381:bool)
        n213 = And(x=w382, y=w381) -> (x .and. y?=w380:bool)
        n214 = case shown="True" w380 {
          frame False {
          }
          frame True {
            n215 = call "Display Message to User5"() -> ()  [unwired: 10 in, 2 out]
            n216 = local write "Begin Run"(FALSE) -> ()
          }
        }
      }
      frame "Shutdown Heat Tape" {
        n217 = local write "Heat Tape"(FALSE) -> ()
        n218 = local write "Circulation Mode"(FALSE) -> ()
      }
      frame "Shutdown Program" {
        w416 = 80.0 ("y")
        n219 = local read "Heat Tape Circulation Out"() -> (w415:dbl)
        n220 = local read "Heat Tape Circulation In"() -> (w417:dbl)
        n221 = Greater?(x=w417, y=w416) -> (0:w413:bool)
        n222 = Greater?(x=w415, y=w416) -> (0:w414:bool)
        n223 = Or(x=w413, y=w414) -> (x .or. y?=w412:bool)
        n224 = case shown="True" w412 {
          tunnel: [T5."Stop" T5."Shutdown Program"] -> w411
          frame False {
            n225 = local write "PD-25 (Circulation Pump)"(FALSE) -> ()
          }
          frame True {
            n226 = local write "PD-25 (Circulation Pump)"(TRUE) -> ()
          }
        }
      }
      frame "Stop" {
        n227 = local write "Emergency Shutdown"(TRUE) -> ()
        n228 = local write "Begin Run"(FALSE) -> ()
        n229 = property on="Login Tab" class="TabCtl (strict)"() -> ("Pages"=w438:refnum<vi>[])  [unwired: 2 in, 2 out]
        n230 = Index Array(array=w438, index=0) -> (element=w440:refnum<vi>)
        n231 = property class="Page"(reference=w440, "PageEnb"=T9."Page Enabled" ("Page Enabled State")) -> (error out=w426:errorcluster)  [unwired: 1 in, 1 out]
        n232 = property on="Login Tab" class="TabCtl (strict)"(error in=w426) -> (error out=w436:errorcluster, "Pages"=w427:refnum<vi>[])  [unwired: 1 in, 1 out]
        n233 = Index Array(array=w427, index=0) -> (element=w429:refnum<vi>)
        n234 = property class="Page"(reference=w429, error in=w436) -> (reference out=w430:refnum<vi>, error out=w437:errorcluster, "PageEnb"=w431:T9)
        n235 = Equal To 0?(x=w431) -> (x = 0?=w432:bool)
        n236 = Select(t=T9."Page Enabled" ("Page Enabled State"), s=w432, f=T9."Page Enabled" ("Page Enabled State")) -> (s? t:f=w435:T9)
        n237 = property class="Page"(reference=w430, error in=w437, "PageEnb"=w435) -> (error out=w425:errorcluster)  [unwired: 1 out]
        n238 = call <vilib>:"Simple Error Handler.vi"("error in (no error)"=w425) -> ()  [unwired: 4 in, 5 out]
      }
    }
  }
  n239 = local write "Login Tab"(enum32{"Login", "Data Aquisition"}."Login" ("Tab Control 3")) -> ()
  n240 = local write "Circulation Run-Time"("0  00:00:00" ("Circulation Run-Time")) -> ()
  n241 = local write "Select Surface"("Select Surface") -> ()
  n242 = local write "Operator Name"("Operator Name") -> ()
  n243 = case shown="False" "Close Camera" {
    tunnel: w4 -> [_ w445]
    tunnel: w3 -> [_ w444]
    frame False {
    }
    frame True {
      n244 = call <vilib>:"IMAQdx Close Camera.vi"("error in"=w444, "Session In"=w445) -> ("error out"=w443:errorcluster)  [unwired: 9 in]
      n245 = call <vilib>:"Simple Error Handler.vi"("error in (no error)"=w443) -> ()  [unwired: 4 in, 5 out]
    }
  }
  "Surface Selected" <- ""
  "Path" <- path "" ("Path")
  "Live View" <- TRUE
